vi "ex_TdmPathToTdxPath.vi"(1 "TDM path":path) -> (0 "TDX path":path)   [LabVIEW 2017]
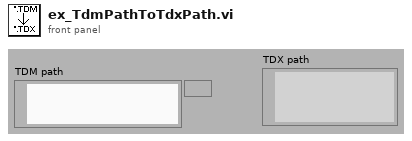
[diagram p1: front panel]
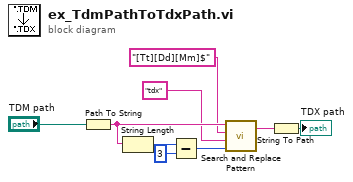
[diagram p0: block diagram]
diagram:
  n1 = Path To String(path="TDM path") -> (string=w4:string)
  n2 = String Length(string=w4) -> (length=w5:i32)
  n3 = Subtract(x=w5, y=3) -> (x-y=w7:i32)
  n4 = call <vilib>:"Search and Replace Pattern.vi"("string"=w4, "regular expression (\"\")"="[Tt][Dd][Mm]$" ("regular expression (\"\")"), "replace string (\"\")"="tdx" ("replace string (\"\")"), "offset (0)"=w7) -> ("result string"=w8:string)  [unwired: 2 out]
  n5 = String To Path(string=w8) -> (path=→"TDX path":path)
